vi "multimetro.vi"() -> (1 "100 misure":string[](array[string]))   [LabVIEW 2013]
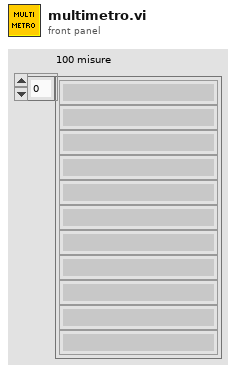
[diagram p1: front panel]
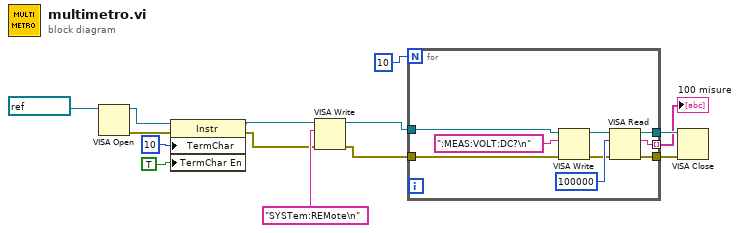
[diagram p0: block diagram]
diagram:
  n1 = VISA Open(VISA resource name=refnum<visa-resource-name> "COM3") -> (VISA resource name=w11:refnum<visa-resource-name>, error out=w10:errorcluster)  [unwired: 4 in]
  n2 = property class="Instr"(reference=w11, error in=w10, "TermChar"=u8 10 ("Message Based Settings:Termination Character"), "TermChar En"=TRUE ("Message Based Settings:Termination Character Enable")) -> (reference out=w4:refnum<visa-resource-name>, error out=w3:errorcluster)
  n3 = VISA Write(VISA resource name=w4, write buffer="SYSTem:REMote\n", error in (no error)=w3) -> (VISA resource name out=w2:refnum<visa-resource-name>, error out=w1:errorcluster)  [unwired: 1 out]
  n4 = for {
    N: 10 -> [_]
    tunnel: w2 -> [w23]
    tunnel: w1 -> [w22]
    tunnel: [w18] -> w9
    tunnel: [w17] -> w8
    tunnel: [w16] -> w7 mode=indexing
    n5 = VISA Write(VISA resource name=w23, write buffer=":MEAS:VOLT:DC?\n", error in (no error)=w22) -> (VISA resource name out=w20:refnum<visa-resource-name>, error out=w15:errorcluster)  [unwired: 1 out]
    n6 = VISA Read(VISA resource name=w20, byte count=u32 100000, error in (no error)=w15) -> (VISA resource name out=w18:refnum<visa-resource-name>, read buffer=w16:string, error out=w17:errorcluster)  [unwired: 1 out]
  }
  "100 misure" <- w7
  n7 = VISA Close(VISA resource name=w9, error in (no error)=w8) -> ()  [unwired: 1 out]
